vi "Teleop.vi"(10 "Match Info":T1={"Autonomous Elapsed Seconds"=0.0, "TeleOp Elapsed Seconds"=0.0, "Disabled Elapsed Seconds"=0.0, "Visited Autonomous"=FALSE, "Visited TeleOp"=FALSE, "Visited Disabled"=FALSE, "Autonomous Settings"={"Autonomous Style"=enum."Independent", "VI Refnum"=refnum}}, 11 "Call Context":T2) -> ()   [LabVIEW 2013]
doc: "This VI is called for each TeleOp packet received from the DS where the robot is not disabled. It is often used to read from the joysticks and update I/O or to update setpoints for timed control loops. It should complete and return within 20 milliseconds or it may miss DS packets."
uses:
  <vilib>/Rock Robotics/WPI/DriverStation/WPI_DriverStationDerivedRobotMode.ctl
  <vilib>/Rock Robotics/WPI/DriverStation/WPI_DriverStationMatch Info.ctl
  <vilib>/Rock Robotics/WPI/Solenoid/WPI_SolenoidValue.ctl
  Robot Global Data.vi
  <vilib>/Rock Robotics/WPI/Solenoid/Deprecated/WPI_SolenoidGetBool.vi
  <vilib>/Rock Robotics/WPI/Solenoid/WPI_SolenoidSetEnum.vi
  <vilib>/Rock Robotics/WPI/Joystick/WPI_JoystickGetSetRefNum.vi
  <vilib>/Rock Robotics/WPI/RobotDrive/WPI_RobotDriveGetSetRefNum.vi
panel:
  out "Voltage":dbl
  out "Value":bool
  out "Ultrasoic Value":dbl
  out "Numeric 1":dbl(slide) scale=0.0..100.0
  out "Boolean 2":bool
  out "Boolean 1":bool
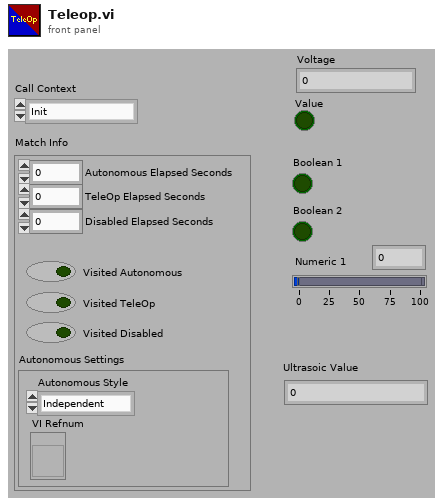
[diagram p1: front panel]
types:
  T1 = typedef "WPI_DriverStationMatch Info.ctl" = cluster{"Autonomous Elapsed Seconds":dbl, "TeleOp Elapsed Seconds":dbl, "Disabled Elapsed Seconds":dbl, "Visited Autonomous":bool, "Visited TeleOp":bool, "Visited Disabled":bool, "Autonomous Settings":cluster{"Autonomous Style":enum16{"Iterative", "Independent"}, "VI Refnum":refnum<vi>}}
  T2 = typedef "WPI_DriverStationDerivedRobotMode.ctl" = enum16{"Init", "Execute", "Stop"}
  T3 = typedef "WPI_AnalogChannelDevRef.ctl" = cluster{"DevStatus":errorcluster, "Analog Module":T4, "Analog Channel":T5}
  T4 = typedef "FPGA_TypedefAnalogModule.ctl" = enum16{"Analog Module 1", "Analog Module 2"}
  T5 = typedef "FPGA_AIChannel.ctl" = enum8{"AI 1", "AI 2", "AI 3", "AI 4", "AI 5", "AI 6", "AI 7", "AI 8", "Invalid"}
  T6 = typedef "WPI_JoystickDevRef.ctl" = cluster{"Device":T7}
  T7 = typedef "WPI_JoystickDeviceEnum.ctl" = enum16{"USB 1", "USB 2", "USB 3", "USB 4", "Kinect 1", "Kinect 2"}
  T8 = typedef "WPI_JoystickButtonState.ctl" = cluster{"Button 1":bool, "Button 2":bool, "Button 3":bool, "Button 4":bool, "Button 5":bool, "Button 6":bool, "Button 7":bool, "Button 8":bool, "Button 9":bool, "Button 10":bool, "Button 11":bool, "Button 12":bool}
  T9 = cluster{"axis 1 (x)":dbl, "axis 2 (y)":dbl, "axis 3 (throttle)":dbl, "axis 4":dbl, "axis 5":dbl, "axis 6":dbl}
  T10 = typedef "WPI_RelayDevRef.ctl" = cluster{"DevStatus":errorcluster, "Relay Channel":T11, "Digital Module":T12, "Relay Direction":T13}
  T11 = typedef "FPGA_DIORelayChannel.ctl" = enum8{"Relay 1", "Relay 2", "Relay 3", "Relay 4", "Relay 5", "Relay 6", "Relay 7", "Relay 8", "Invalid"}
  T12 = typedef "FPGA_TypedefDigitalModule.ctl" = enum16{"Digital Module 1", "Digital Module 2"}
  T13 = typedef "WPI_RelayDirection.ctl" = enum16{"Both directions", "Forward only", "Reverse only"}
  T14 = typedef "WPI_RobotDriveDevRef.ctl" = cluster{"DevStatus":errorcluster, "Motors[]":T15[], "Square Inputs":bool, "Max Output":dbl, "Isochronous":bool}
  T15 = typedef "WPI_MotorControlDeviceRef.ctl" = cluster{"DeviceStatus":errorcluster, "Type":enum16{"PWM", "CAN"}, "PWM":cluster{"Digital Module":T12, "PWM Channel":T16, "DeadBand":T17}, "CAN":cluster{"Device Number":u8, "Control Mode":T18, "Semaphore":T19, "Max Vout":dbl}, "Invert":bool, "TransformRef":T20, "InvTransformRef":T20}
  T16 = typedef "FPGA_DIOPWMChannel.ctl" = enum8{"PWM 1", "PWM 2", "PWM 3", "PWM 4", "PWM 5", "PWM 6", "PWM 7", "PWM 8", "PWM 9", "PWM 10", "Invalid"}
  T17 = typedef "WPI_PWMDeadband.ctl" = cluster{"Name":string, "maxPositivePwm":i32, "minPositivePwm":i32, "centerPwm":i32, "maxNegativePwm":i32, "minNegativePwm":i32, "angularRange":u16}
  T18 = typedef "WPI_CANJaguar_ControlMode.ctl" = enum8{"Percent VBus", "Current", "Speed", "Position", "Voltage"}
  T19 = typedef "Semaphore RefNum" = refnum<k1>
  T20 = typedef "WPI_PWMTransform_ConPane.ctl" = refnum<vi>
  T21 = typedef "WPI_DigitalInputDevRef.ctl" = cluster{"DevStatus":errorcluster, "DIO Channel":T22, "Digital Module":T12}
  T22 = typedef "FPGA_DIOChannel.ctl" = enum8{"DIO 1", "DIO 2", "DIO 3", "DIO 4", "DIO 5", "DIO 6", "DIO 7", "DIO 8", "DIO 9", "DIO 10", "DIO 11", "DIO 12", "DIO 13", "DIO 14", "Invalid"}
  T23 = typedef "WPI_SolenoidDevRef.ctl" = cluster{"DevStatus":errorcluster, "Solenoid Module":T24, "Forward Solenoid Channel":T25, "Reverse Solenoid Channel":T25}
  T24 = typedef "FPGA_TypedefSolenoidModule.ctl" = enum16{"Solenoid Module 1", "Solenoid Module 2"}
  T25 = typedef "WPI_SolenoidChannel.ctl" = enum8{"Solenoid 1", "Solenoid 2", "Solenoid 3", "Solenoid 4", "Solenoid 5", "Solenoid 6", "Solenoid 7", "Solenoid 8", "Invalid"}
  T26 = typedef "WPI_SolenoidValue.ctl" = enum16{"Off", "On", "Forward", "Reverse"}
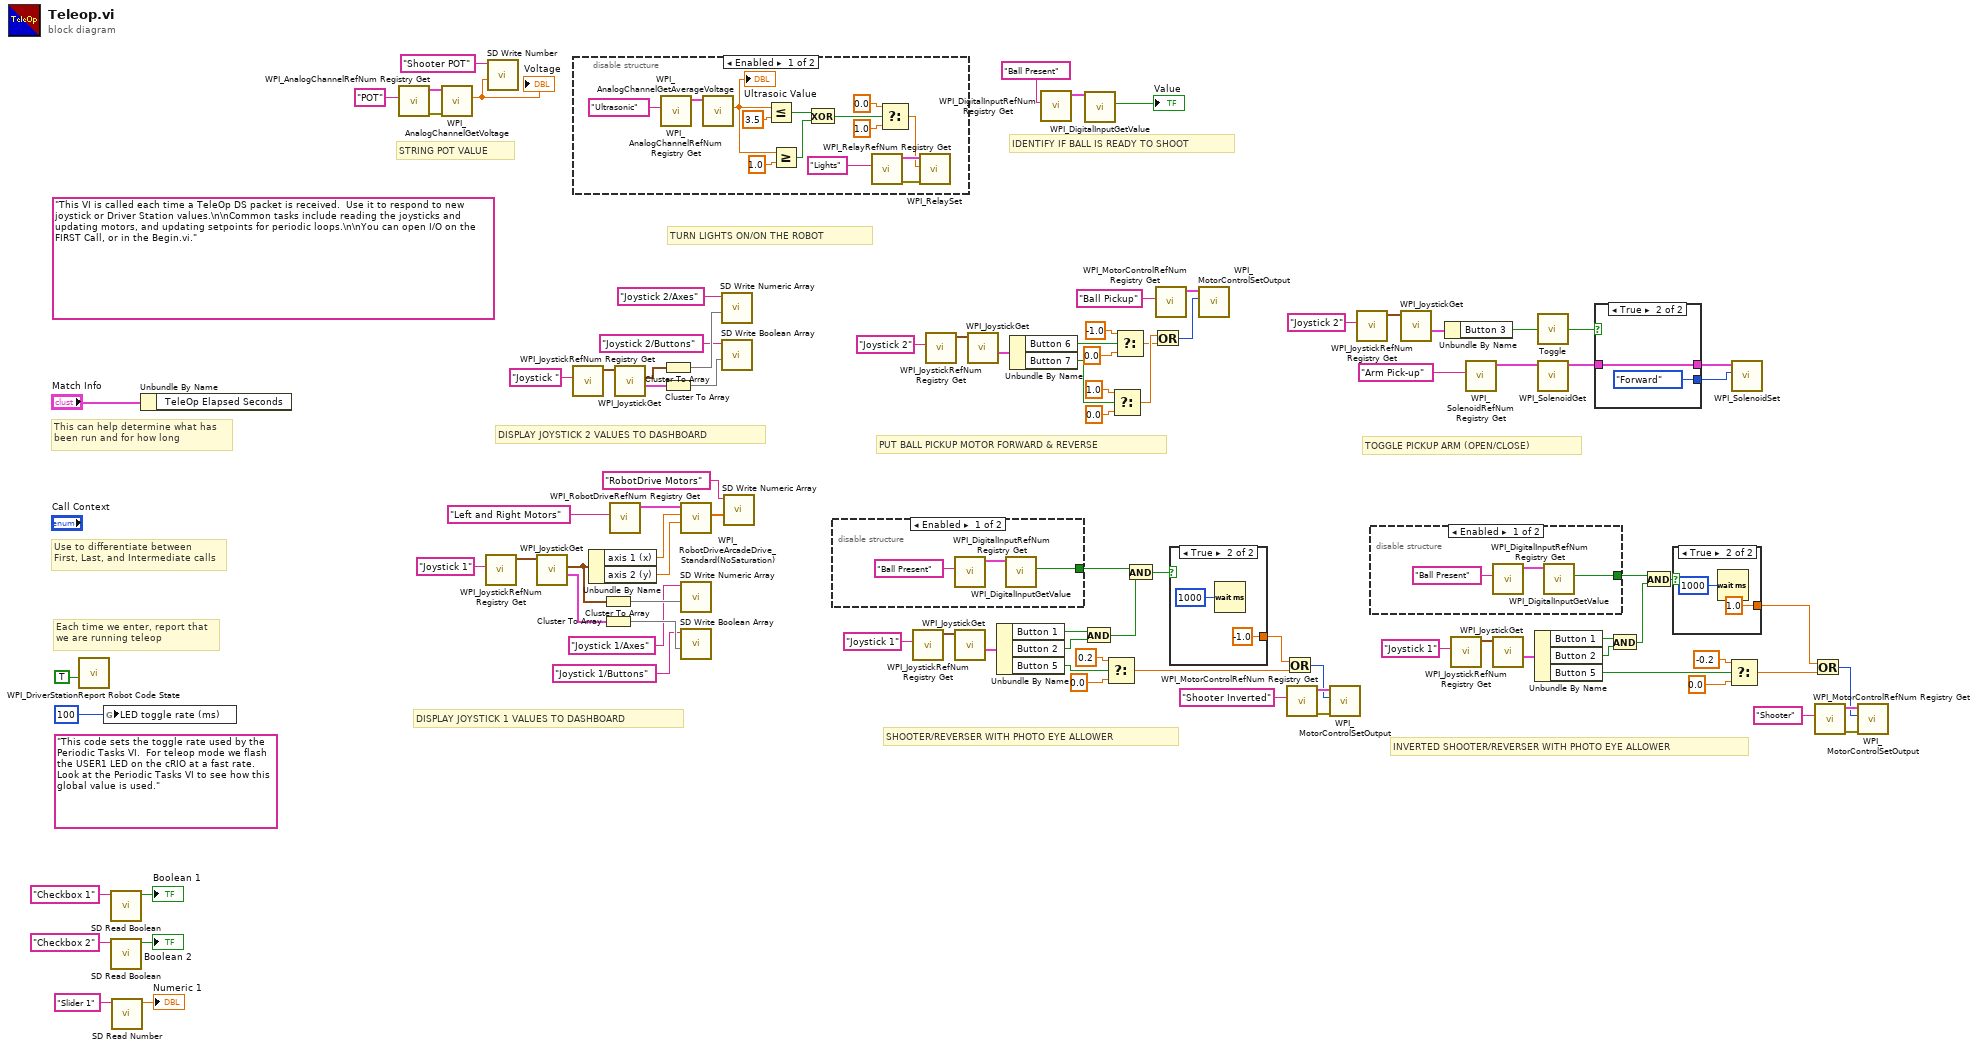
[diagram p0: block diagram]
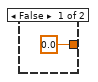
[diagram p2: hidden frame]
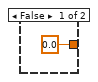
[diagram p3: hidden frame]
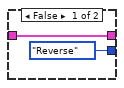
[diagram p7: hidden frame]
diagram:
  (unwired) "This code sets the toggle rate used by the Periodic Tasks VI.  For teleop mode we flash the USER1 LED on the cRIO at a fast rate.  Look at the Periodic Tasks VI to see how this global value is used."
  (unwired) "This VI is called each time a TeleOp DS packet is received.  Use it to respond to new joystick or Driver Station values.\n\nCommon tasks include reading the joysticks and updating motors, and updating setpoints for periodic loops.\n\nYou can open I/O on the FIRST Call, or in the Begin.vi."
  # "INVERTED SHOOTER/REVERSER WITH PHOTO EYE ALLOWER"
  # "SHOOTER/REVERSER WITH PHOTO EYE ALLOWER"
  # "TOGGLE PICKUP ARM (OPEN/CLOSE)"
  # "PUT BALL PICKUP MOTOR FORWARD & REVERSE"
  # "DISPLAY JOYSTICK 1 VALUES TO DASHBOARD"
  # "DISPLAY JOYSTICK 2 VALUES TO DASHBOARD"
  # "IDENTIFY IF BALL IS READY TO SHOOT"
  # "TURN LIGHTS ON/ON THE ROBOT"
  # "STRING POT VALUE"
  # "Each time we enter, report that\nwe are running teleop"
  # "Use to differentiate between\nFirst, Last, and Intermediate calls"
  # "This can help determine what has\nbeen run and for how long"
  n1 = call <vilib>:"WPI_DriverStationReport Robot Code State.vi"("TeleOp"=TRUE ("Autonomous")) -> ()  [unwired: 10 in, 1 out]
  n2 = global write "Robot Global Data.vi" "LED toggle rate (ms)"(u32 100 ("LED ms toggle rate")) -> ()
  n3 = call <vilib>:"SD Read Boolean.vi"("Name"="Checkbox 1" ("refnum name")) -> ("Boolean"=→"Boolean 1":bool)  [unwired: 8 in, 2 out]
  n4 = call <vilib>:"SD Read Boolean.vi"("Name"="Checkbox 2" ("refnum name")) -> ("Boolean"=→"Boolean 2":bool)  [unwired: 8 in, 2 out]
  n5 = call <vilib>:"SD Read Number.vi"("Name"="Slider 1" ("refnum name")) -> ("Numeric"=→"Numeric 1":dbl)  [unwired: 8 in, 2 out]
  n6 = Unbundle By Name("Match Info") -> ()  [unwired: 1 out]
  n7 = call <vilib>:"WPI_AnalogChannelRefNum Registry Get.vi"("refnum name"="POT") -> ("error out"=w34:errorcluster, "AIDeviceRef"=w35:T3)  [unwired: 9 in]
  n8 = call <vilib>:"WPI_AnalogChannelGetVoltage.vi"("error in (no error)"=w34, "AIDeviceRef"=w35) -> ("Voltage"=w32:dbl)  [unwired: 7 in, 2 out]
  "Voltage" <- w32
  n9 = call <vilib>:"WPI_JoystickRefNum Registry Get.vi"("refnum name"="Joystick 1") -> ("JoystickDevRef"=w91:T6)  [unwired: 1 in, 9 out]
  n10 = call <vilib>:"SD Write Number.vi"("Numeric"=w32, "Name"="Shooter POT" ("Table Prefix out")) -> ()  [unwired: 8 in, 2 out]
  n11 = call <vilib>:"WPI_JoystickGet.vi"("JoystickDevRef"=w91) -> ("Buttons"=w88:T8, "Axes"=w85:T9)  [unwired: 1 in, 4 out]
  n12 = call <vilib>:"WPI_JoystickRefNum Registry Get.vi"("refnum name"="Joystick ") -> ("JoystickDevRef"=w24:T6)  [unwired: 1 in, 9 out]
  n13 = disable-structure shown="Enabled" {
    frame Enabled {
      n14 = call <vilib>:"WPI_AnalogChannelRefNum Registry Get.vi"("refnum name"="Ultrasonic") -> ("AIDeviceRef"=w110:T3)  [unwired: 9 in, 1 out]
      n15 = call <vilib>:"WPI_AnalogChannelGetAverageVoltage.vi"("AIDeviceRef"=w110) -> ("Voltage"=w109:dbl)  [unwired: 8 in, 2 out]
      "Ultrasoic Value" <- w109
      n16 = Less Or Equal?(x=w109, y=3.5) -> (x <= y?=w106:bool)
      n17 = Greater Or Equal?(x=w109, y=1.0) -> (x >= y?=w105:bool)
      n18 = Exclusive Or(1:w105, 2:w106) -> (0:w104:bool)
      n19 = call <vilib>:"WPI_RelayRefNum Registry Get.vi"("refnum name"="Lights") -> ("error out"=w101:errorcluster, "RelayDevRef"=w100:T10)  [unwired: 9 in]
      n20 = Select(t=0.0, s=w104, f=1.0) -> (s? t:f=w99:dbl)
      n21 = call <vilib>:"WPI_RelaySet.vi"("error in (no error)"=w101, "RelayValue"=w99, "RelayDevRef"=w100) -> ()  [unwired: 7 in, 2 out]
    }
    frame Disabled {
    }
  }
  n22 = Unbundle By Name(w85) -> ("axis 1 (x)"=w94:dbl, "axis 2 (y)"=w93:dbl)
  n23 = Cluster To Array(cluster=w85) -> (array=w84:dbl[])
  n24 = Cluster To Array(cluster=w88) -> (array=w87:bool[])
  n25 = call <vilib>:"WPI_RobotDriveRefNum Registry Get.vi"("refnum name"="Left and Right Motors") -> ("RobotDriveDevRef"=w95:T14)  [unwired: 1 in, 9 out]
  n26 = call <vilib>:"WPI_JoystickGet.vi"("JoystickDevRef"=w24) -> ("Buttons"=w25:T8, "Axes"=w28:T9)  [unwired: 1 in, 4 out]
  n27 = Cluster To Array(cluster=w28) -> (array=w29:dbl[])
  n28 = Cluster To Array(cluster=w25) -> (array=w26:bool[])
  n29 = call <vilib>:"WPI_RobotDriveArcadeDrive_Standard(NoSaturation).vi"("Y axis value"=w93, "X axis value"=w94, "RobotDriveDevRef"=w95) -> ("Motor Values"=w81:dbl[])  [unwired: 1 in, 7 out]
  n30 = call <vilib>:"SD Write Numeric Array.vi"("Numeric Array"=w84, "Name"="Joystick 1/Axes") -> ()  [unwired: 8 in, 2 out]
  n31 = call <vilib>:"SD Write Boolean Array.vi"("Boolean Array"=w87, "Name"="Joystick 1/Buttons") -> ()  [unwired: 8 in, 2 out]
  n32 = call <vilib>:"SD Write Numeric Array.vi"("Numeric Array"=w29, "Name"="Joystick 2/Axes") -> ()  [unwired: 8 in, 2 out]
  n33 = call <vilib>:"SD Write Boolean Array.vi"("Boolean Array"=w26, "Name"="Joystick 2/Buttons") -> ()  [unwired: 8 in, 2 out]
  n34 = call <vilib>:"SD Write Numeric Array.vi"("Numeric Array"=w81, "Name"="RobotDrive Motors") -> ()  [unwired: 8 in, 2 out]
  n35 = disable-structure shown="Enabled" {
    disable-tunnel: [w112 _] -> w9
    frame Enabled {
      n36 = call <vilib>:"WPI_DigitalInputRefNum Registry Get.vi"("refnum name"="Ball Present") -> ("DigitalInputDevRef"=w113:T21)  [unwired: 9 in, 1 out]
      n37 = call <vilib>:"WPI_DigitalInputGetValue.vi"("DigitalInputDevRef"=w113) -> ("Value"=w112:bool)  [unwired: 8 in, 2 out]
    }
    frame Disabled {
    }
  }
  n38 = call <vilib>:"WPI_JoystickRefNum Registry Get.vi"("refnum name"="Joystick 1") -> ("JoystickDevRef"=w67:T6)  [unwired: 9 in, 1 out]
  n39 = call <vilib>:"WPI_JoystickRefNum Registry Get.vi"("refnum name"="Joystick 2") -> ("JoystickDevRef"=w57:T6)  [unwired: 9 in, 1 out]
  n40 = call <vilib>:"WPI_JoystickGet.vi"("JoystickDevRef"=w67) -> ("Buttons"=w68:T8)  [unwired: 4 in, 2 out]
  n41 = call <vilib>:"WPI_JoystickGet.vi"("JoystickDevRef"=w57) -> ("Buttons"=w58:T8)  [unwired: 4 in, 2 out]
  n42 = Unbundle By Name(w68) -> ("Button 1"=w40:bool, "Button 2"=w41:bool, "Button 5"=w5:bool)
  n43 = Unbundle By Name(w58) -> ("Button 6"=w59:bool, "Button 7"=w55:bool)
  n44 = call <vilib>:"WPI_DigitalInputRefNum Registry Get.vi"("refnum name"="Ball Present") -> ("DigitalInputDevRef"=w21:T21)  [unwired: 9 in, 1 out]
  n45 = And(x=w40, y=w41) -> (x .and. y?=w10:bool)
  n46 = call <vilib>:"WPI_DigitalInputGetValue.vi"("DigitalInputDevRef"=w21) -> ("Value"=→"Value":bool)  [unwired: 8 in, 2 out]
  n47 = Select(t=0.2, s=w5, f=0.0) -> (s? t:f=w3:dbl)
  n48 = Select(t=1.0, s=w55, f=0.0) -> (s? t:f=w54:dbl)
  n49 = Select(t=-1.0, s=w59, f=0.0) -> (s? t:f=w53:dbl)
  n50 = And(x=w9, y=w10) -> (x .and. y?=w8:bool)
  n51 = Or(x=w54, y=w53) -> (x .or. y?=w52:i32)
  n52 = call <vilib>:"WPI_MotorControlRefNum Registry Get.vi"("refnum name"="Ball Pickup") -> ("MotorControlDevRef"=w64:T15)  [unwired: 9 in, 1 out]
  n53 = case shown="True" w8 {
    tunnel: [0.0 -1.0] -> w4
    frame False {
    }
    frame True {
      n54 = Wait (ms)(milliseconds to wait=u32 1000) -> ()  [unwired: 1 out]
    }
  }
  n55 = call <vilib>:"WPI_MotorControlSetOutput.vi"("Output"=w52, "MotorControlDevRef"=w64) -> ()  [unwired: 7 in, 3 out]
  n56 = Or(x=w4, y=w3) -> (x .or. y?=w2:i32)
  n57 = call <vilib>:"WPI_MotorControlRefNum Registry Get.vi"("refnum name"="Shooter Inverted") -> ("error out"=w37:errorcluster, "MotorControlDevRef"=w38:T15)  [unwired: 9 in]
  n58 = call <vilib>:"WPI_MotorControlSetOutput.vi"("error in (no error)"=w37, "Output"=w2, "MotorControlDevRef"=w38) -> ()  [unwired: 6 in, 3 out]
  n59 = call <vilib>:"WPI_JoystickRefNum Registry Get.vi"("refnum name"="Joystick 2") -> ("JoystickDevRef"=w49:T6)  [unwired: 9 in, 1 out]
  n60 = disable-structure shown="Enabled" {
    disable-tunnel: [w118 _] -> w19
    frame Enabled {
      n61 = call <vilib>:"WPI_DigitalInputRefNum Registry Get.vi"("refnum name"="Ball Present") -> ("DigitalInputDevRef"=w120:T21)  [unwired: 9 in, 1 out]
      n62 = call <vilib>:"WPI_DigitalInputGetValue.vi"("DigitalInputDevRef"=w120) -> ("Value"=w118:bool)  [unwired: 8 in, 2 out]
    }
    frame Disabled {
    }
  }
  n63 = call <vilib>:"WPI_JoystickGet.vi"("JoystickDevRef"=w49) -> ("Buttons"=w48:T8)  [unwired: 4 in, 2 out]
  n64 = Unbundle By Name(w48) -> ("Button 3"=w42:bool)
  n65 = call <vilib>:"WPI_JoystickRefNum Registry Get.vi"("refnum name"="Joystick 1") -> ("JoystickDevRef"=w73:T6)  [unwired: 9 in, 1 out]
  n66 = call <vilib>:"WPI_SolenoidRefNum Registry Get.vi"("refnum name"="Arm Pick-up") -> ("SolenoidDevRef"=w47:T23)  [unwired: 9 in, 1 out]
  n67 = call <vilib>:"WPI_JoystickGet.vi"("JoystickDevRef"=w73) -> ("Buttons"=w72:T8)  [unwired: 4 in, 2 out]
  n68 = Unbundle By Name(w72) -> ("Button 1"=w39:bool, "Button 2"=w17:bool, "Button 5"=w13:bool)
  n69 = call "Toggle.vi"("Input"=w42) -> ("Toggled Output"=w46:bool)
  n70 = call-poly <vilib>:"WPI_SolenoidGet.vi"("SolenoidDevRef"=w47) -> ("SolenoidDevRef"=w45:T23)  [unwired: 8 in, 2 out]
  n71 = case shown="True" w46 {
    tunnel: w45 -> [w122 w124]
    tunnel: [w122 w124] -> w44
    tunnel: [WPI_SolenoidValue."Reverse" ("Value") WPI_SolenoidValue."Forward" ("Value")] -> w43
    frame False {
    }
    frame True {
    }
  }
  n72 = And(x=w39, y=w17) -> (x .and. y?=w18:bool)
  n73 = And(x=w19, y=w18) -> (x .and. y?=w16:bool)
  n74 = case shown="True" w16 {
    tunnel: [0.0 1.0] -> w12
    frame False {
    }
    frame True {
      n75 = Wait (ms)(milliseconds to wait=u32 1000) -> ()  [unwired: 1 out]
    }
  }
  n76 = Select(t=-0.2, s=w13, f=0.0) -> (s? t:f=w11:dbl)
  n77 = call-poly <vilib>:"WPI_SolenoidSet.vi"("Value"=w43, "SolenoidDevRef"=w44) -> ()  [unwired: 8 in, 2 out]
  n78 = Or(x=w12, y=w11) -> (x .or. y?=w1:i32)
  n79 = call <vilib>:"WPI_MotorControlRefNum Registry Get.vi"("refnum name"="Shooter") -> ("error out"=w70:errorcluster, "MotorControlDevRef"=w69:T15)  [unwired: 9 in]
  n80 = call <vilib>:"WPI_MotorControlSetOutput.vi"("error in (no error)"=w70, "Output"=w1, "MotorControlDevRef"=w69) -> ()  [unwired: 6 in, 3 out]
